vi "CanBurglerControl.vi"(8 "error in (no error)":errorcluster, 11 "Robot Commands":T1) -> (0 "error out":errorcluster)   [LabVIEW 2014]
uses:
  Joystick/Robot Commands.ctl
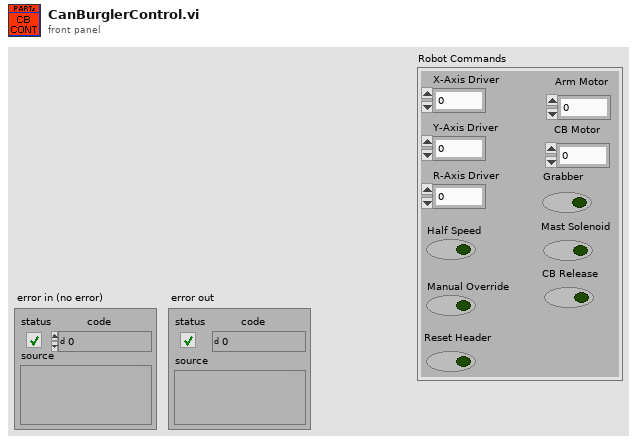
[diagram p1: front panel]
types:
  T1 = typedef "Robot Commands.ctl" = cluster{"X-Axis Driver":dbl, "Y-Axis Driver":dbl, "R-Axis Driver":dbl, "Half Speed":bool, "Manual Override":bool, "Reset Header":bool, "Arm Motor":dbl, "CB Motor":dbl, "Grabber":bool, "Mast Solenoid":bool, "CB Release":bool}
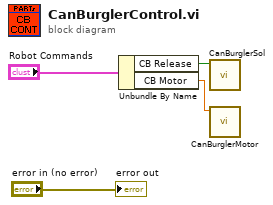
[diagram p0: block diagram]
diagram:
  n1 = Unbundle By Name("Robot Commands") -> ("CB Release"=w3:bool, "CB Motor"=w2:dbl)
  n2 = call "CanBurglerSol.vi"("Grabber Open/Close"=w3) -> ()  [unwired: 10 in, 1 out]
  n3 = call "CanBurglerMotor.vi"("Output"=w2) -> ()  [unwired: 10 in, 1 out]
  "error out" <- "error in (no error)"
